vi "Get Fabic Style Atributes.vi"(1 "connectString":string, 2 "Ring Refnum":refnum<vi>) -> (0 "projectileAttribs":T1)   [LabVIEW 2012]
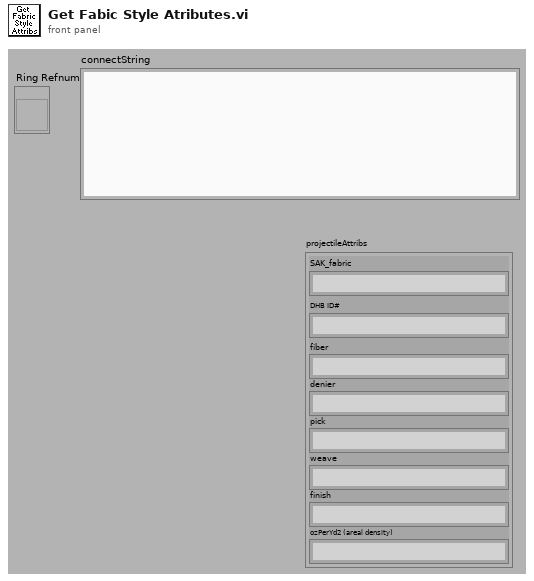
[diagram p1: front panel]
types:
  T1 = cluster{"fiber":string, "denier":string, "pick":string, "weave":string, "finish":string, "ozPerYd2":string, "fabricStyle_DHB":string, "fabricStyle_DHB 2":string}
  T2 = cluster{"recordset data[0]":string, "recordset data[1]":string, "recordset data[2]":string, "recordset data[3]":string, "recordset data[4]":string, "recordset data[5]":string, "recordset data[6]":string, "recordset data[7]":string}
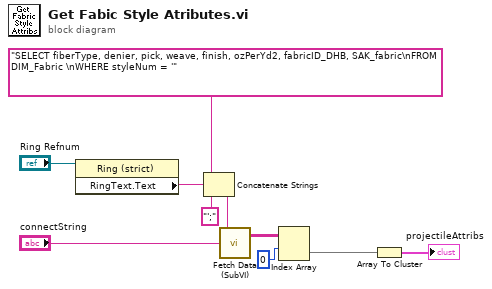
[diagram p0: block diagram]
diagram:
  n1 = property on="Property Node" class="Ring (strict)"(reference="Ring Refnum") -> ("RingText.Text"=w2:string)  [unwired: 1 in, 2 out]
  n2 = Concatenate Strings("SELECT fiberType, denier, pick, weave, finish, ozPerYd2, fabricID_DHB, SAK_fabric\nFROM DIM_Fabric \nWHERE styleNum = '", w2, "';" ("string")) -> (w5:string)
  n3 = call "Fetch Data (SubVI).vi"("connectString"="connectString", "query string"=w5) -> ("recordset data"=w10:string[][])  [unwired: 1 in, 1 out]
  n4 = Index Array(array=w10, index (row)=0 ("disabled index (col)")) -> (element=w1:string[])  [unwired: 1 in]
  n5 = Array To Cluster(array=w1) -> (cluster=→"projectileAttribs":T2)
